vi "Execute.vi"(8 "error in (no error)":errorcluster, 9 "Workspace":T1, 10 "Cluster":T2, 11 "Pick and Place in":refnum<class "Pick and Place.lvclass">) -> (0 "error out":errorcluster, 2 "Control Out":T2, 3 "Pick and Place out":refnum<class "Pick and Place.lvclass">)   [LabVIEW 2020, in "Pick and Place.lvclass"]
uses:
  Pick and Place.lvclass
  Controller/Controllers.ctl
  Controller/I-O/I-O.lvclass
  Controller/Dispenser/Dispenser.lvclass
  C:/Program Files (x86)/Aerotech/A3200/LabVIEW/2010/Bin/Aerotech.A3200.dll
  Program Files (x86)/Aerotech/A3200/LabVIEW/2010/Bin/Aerotech.A3200.dll
  Workspace/Workspace.ctl
  Pick and Place.lvclass/Pick and Place.ctl
  686f831b-46dc-4046-ae8d-e6191224ee14.vi
  Controller/Motion/Motion.lvclass
  Controller/Motion/A3200/A3200.lvclass
  Controller/Controller.lvclass
  Workspace/Fixture.lvclass
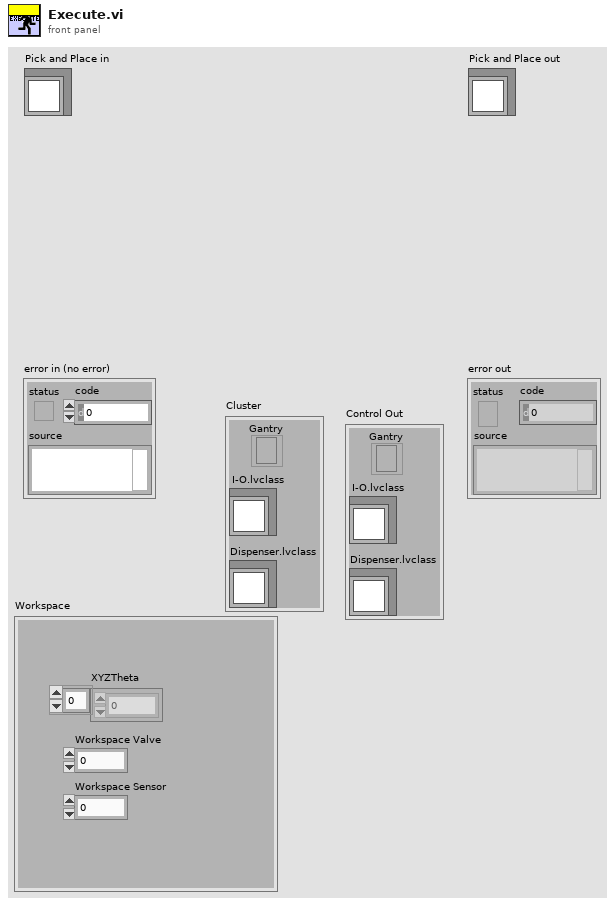
[diagram p1: front panel]
types:
  T1 = typedef "Fixture.lvclass/Workspace.ctl" = cluster{"XYZTheta":dbl[], "Workspace Valve":i32, "Workspace Sensor":i32}
  T2 = typedef "Controller.lvclass/Controllers.ctl" = cluster{"I-O.lvclass":refnum<class "I-O.lvclass">, "Dispenser.lvclass":refnum<class "Dispenser.lvclass">, "Gantry":refnum<k24>}
  T3 = typedef "Pick and Place.lvclass/Pick and Place Type.ctl" = enum16{"Primary Pick Up", "Secondary Pick Up", "Put Down All", "Pick Up All", "Put Down Secondary"}
  T4 = typedef "I-O.lvclass/Pin Map.ctl" = cluster{"Region Valves":i32[], "Extra Valves":dbl[][][], "Tool Primary Valve":i32, "Tool Secondary Valve":i32, "Region Sensors":i32[], "Extra Sensors":dbl[][][], "Tool Primary Sensor":dbl, "Tool Secondary Sensor":dbl, "Compression Sensor":dbl, "5V":i32}
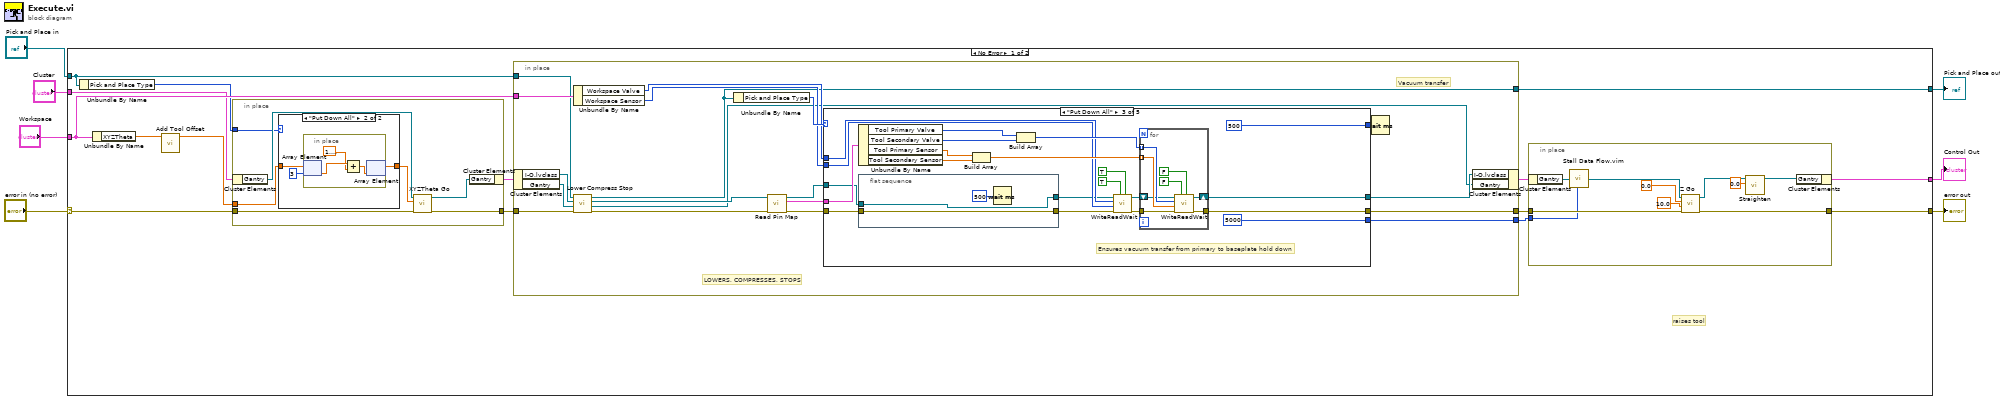
[diagram p0: block diagram]
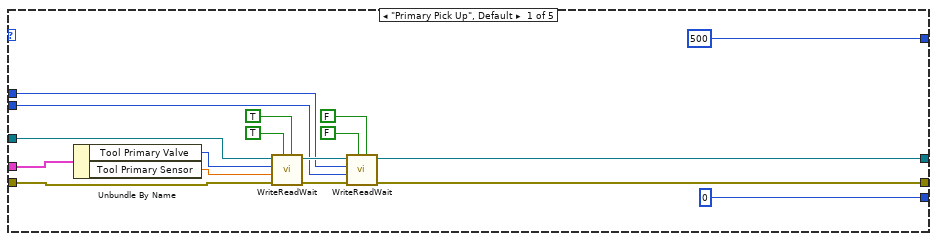
[diagram p2: hidden frame]
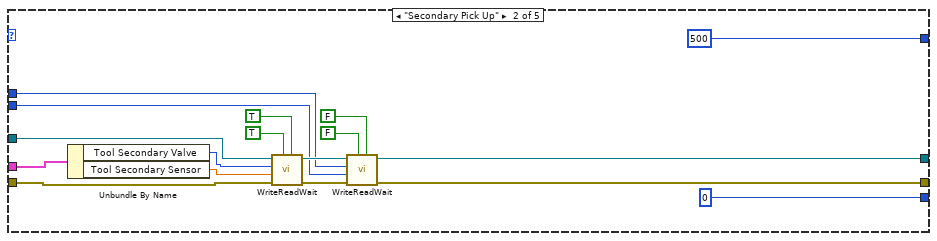
[diagram p3: hidden frame]
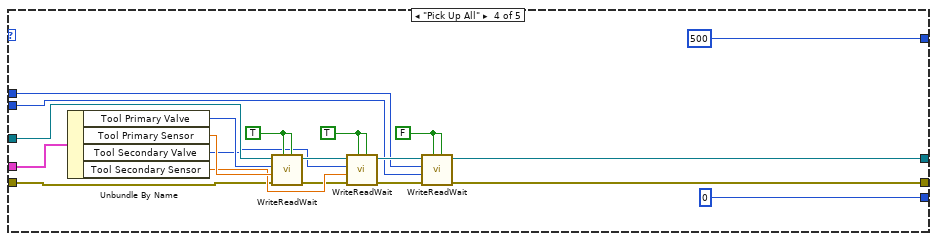
[diagram p4: hidden frame]
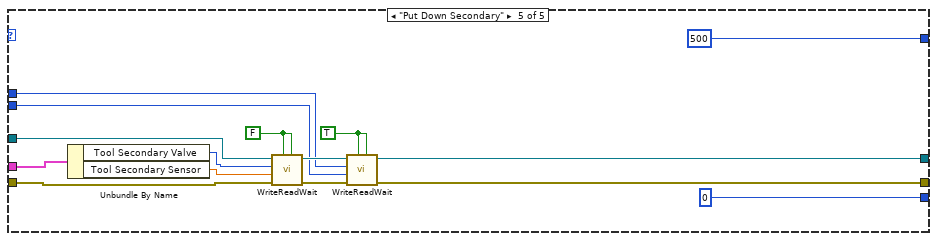
[diagram p5: hidden frame]
diagram:
  n1 = case shown="No Error" "error in (no error)" {
    selector: "error in (no error)" -> [w16 w168]
    tunnel: "Cluster" -> [w20 w169]
    tunnel: "Workspace" -> [w21 _]
    tunnel: [w15 w168] -> w1
    tunnel: [w19 w169] -> w2
    tunnel: "Pick and Place in" -> [w9 w167]
    tunnel: [w18 w167] -> w6
    frame No Error {
      # "raises tool"
      n2 = Unbundle By Name(w9) -> ("Pick and Place Type"=w8:T3)
      n3 = Unbundle By Name(w21) -> ("XYZTheta"=w13:dbl[])
      n4 = call "Add Tool Offset.vi"("XYZTheta"=w13) -> ("Array"=w17:dbl[])  [unwired: 10 in]
      n5 = in-place {
        in-place-border: w17 -> [w154]
        in-place-border: w16 -> [w156]
        in-place-border: [w157] -> w12
        in-place-border: w8 -> [w155]
        n6 = in-place-cluster #1(w20) -> ("Gantry"=w159:refnum<k24>)
        n7 = case shown="\"Put Down All\"" w155 {
          tunnel: w154 -> [w160 w163]
          tunnel: [w160 w161] -> w153
          frame "Primary Pick Up", Default {
          }
          frame "Put Down All" {
            n8 = in-place {
              n9 = in-place-array #2(w163, 3) -> (w166:dbl)
              n10 = Add(x=w166, y=1.5707963267948966) -> (x+y=w164:dbl)
              n11 = in-place-array #2(w164) -> (w161:dbl[])  [unwired: 1 out]
            }
          }
        }
        n12 = call "XYZTheta Go.vi"("error in (no error)"=w156, "XYZTheta In"=w153, "Gantry 2"=w159) -> ("error out"=w157:errorcluster, "Gantry 3"=w158:refnum<k24>)  [unwired: 6 in, 1 out]
        n13 = in-place-cluster #1("Gantry"=w158) -> (w22:T2)
      }
      n14 = in-place {
        in-place-border: w21 -> [w51]
        in-place-border: w9 -> [w41]
        in-place-border: [w40] -> w18
        in-place-border: w12 -> [w35]
        in-place-border: [w34] -> w11
        in-place-border: [w33] -> w10
        # "Vacuum transfer"
        # "LOWERS, COMPRESSES, STOPS"
        n15 = in-place-cluster #3(w22) -> ("I-O.lvclass"=w44:refnum<class "I-O.lvclass">, "Gantry"=w39:refnum<k24>)
        n16 = Unbundle By Name(w51) -> ("Workspace Valve"=w49:i32, "Workspace Sensor"=w48:i32)
        n17 = call "Lower Compress Stop.vi"("error in (no error)"=w35, "Gantry In"=w39, "I-O.lvclass"=w44, "Pick and Place in"=w41) -> ("error out"=w37:errorcluster, "Gantry Out"=w38:refnum<k24>, "I-O out"=w42:refnum<class "I-O.lvclass">, "Pick and Place Out"=w40:refnum<class "Pick and Place.lvclass">)  [unwired: 4 in]
        n18 = Unbundle By Name(w40) -> ("Pick and Place Type"=w50:T3)
        n19 = call-dynamic "Read Pin Map.vi"("error in (no error)"=w37, "I-O in"=w42) -> ("error out"=w36:errorcluster, "Pin Map 2"=w46:T4, "I-O out"=w45:refnum<class "I-O.lvclass">)  [unwired: 7 in]
        n20 = case shown="\"Put Down All\"" w50 {
          tunnel: w49 -> [w65 w77 w96 w127 w146]
          tunnel: w48 -> [w64 w76 w95 w126 w145]
          tunnel: [w59 w75 w100 w124 w143] -> w43
          tunnel: [u32 500 ("milliseconds to wait") 500 500 u32 500 ("milliseconds to wait") u32 500 ("milliseconds to wait")] -> w47
          tunnel: w45 -> [w58 w74 w91 w136 w151]
          tunnel: w46 -> [w57 w73 w94 w137 w152]
          tunnel: w36 -> [w55 w72 w88 w122 w141]
          tunnel: [w53 w70 w87 w119 w139] -> w34
          tunnel: [0 0 5000 0 0] -> w33
          frame "Primary Pick Up", Default {
            n21 = Unbundle By Name(w57) -> ("Tool Primary Valve"=w56:i32, "Tool Primary Sensor"=w67:dbl)
            n22 = call "WriteReadWait.vi"("Read Value"=TRUE, "Write Value"=TRUE, "error in (no error)"=w55, "Read"=w67, "Write"=w56, "I-O in"=w58) -> ("error out"=w54:errorcluster, "I-O out"=w66:refnum<class "I-O.lvclass">)  [unwired: 4 in]
            n23 = call "WriteReadWait.vi"("Read Value"=FALSE ("Write Value"), "Write Value"=FALSE ("Read Value"), "error in (no error)"=w54, "Read"=w64, "Write"=w65, "I-O in"=w66) -> ("error out"=w53:errorcluster, "I-O out"=w59:refnum<class "I-O.lvclass">)  [unwired: 4 in]
          }
          frame "Secondary Pick Up" {
            n24 = Unbundle By Name(w73) -> ("Tool Secondary Valve"=w79:i32, "Tool Secondary Sensor"=w78:dbl)
            n25 = call "WriteReadWait.vi"("Read Value"=TRUE, "Write Value"=TRUE, "error in (no error)"=w72, "Read"=w78, "Write"=w79, "I-O in"=w74) -> ("error out"=w71:errorcluster, "I-O out"=w84:refnum<class "I-O.lvclass">)  [unwired: 4 in]
            n26 = call "WriteReadWait.vi"("Read Value"=FALSE ("Write Value"), "Write Value"=FALSE ("Read Value"), "error in (no error)"=w71, "Read"=w76, "Write"=w77, "I-O in"=w84) -> ("error out"=w70:errorcluster, "I-O out"=w75:refnum<class "I-O.lvclass">)  [unwired: 4 in]
          }
          frame "Put Down All" {
            # "Ensures vacuum transfer from primary to baseplate hold down"
            n27 = Unbundle By Name(w94) -> ("Tool Primary Valve"=w101:i32, "Tool Secondary Valve"=w102:i32, "Tool Primary Sensor"=w103:dbl, "Tool Secondary Sensor"=w104:dbl)
            n28 = flat-sequence {
              tunnel: [w108] -> w92
              tunnel: w91 -> [w108]
              tunnel: [w107] -> w89
              tunnel: w88 -> [w107]
              frame #0 {
                # "Delay After Placing"
                n29 = Wait (ms)(milliseconds to wait=u32 500) -> ()  [unwired: 1 out]
              }
            }
            n30 = Build Array(w103, w104) -> (w106:dbl[])
            n31 = Build Array(w101, w102) -> (w105:i32[])
            n32 = call "WriteReadWait.vi"("Read Value"=TRUE, "Write Value"=TRUE, "error in (no error)"=w89, "Read"=w95, "Write"=w96, "I-O in"=w92) -> ("error out"=w90:errorcluster, "I-O out"=w93:refnum<class "I-O.lvclass">)  [unwired: 4 in]
            n33 = for {
              shift-right: [w112] -> w100
              shift-left: w93 -> [w113]
              tunnel: w105 -> [w115] mode=indexing
              tunnel: w106 -> [w114] mode=indexing
              tunnel: w90 -> [w111]
              tunnel: [w110] -> w87
              n34 = call "WriteReadWait.vi"("Read Value"=FALSE ("Write Value"), "Write Value"=FALSE ("Read Value"), "error in (no error)"=w111, "Read"=w114, "Write"=w115, "I-O in"=w113) -> ("error out"=w110:errorcluster, "I-O out"=w112:refnum<class "I-O.lvclass">)  [unwired: 4 in]
            }
          }
          frame "Pick Up All" {
            w125 = FALSE ("Read Value")
            w129 = TRUE ("Write Value")
            w135 = TRUE ("Write Value")
            n35 = Unbundle By Name(w137) -> ("Tool Primary Valve"=w134:i32, "Tool Primary Sensor"=w133:dbl, "Tool Secondary Valve"=w131:i32, "Tool Secondary Sensor"=w130:dbl)
            n36 = call "WriteReadWait.vi"("Read Value"=w135, "Write Value"=w135, "error in (no error)"=w122, "Read"=w133, "Write"=w134, "I-O in"=w136) -> ("error out"=w121:errorcluster, "I-O out"=w132:refnum<class "I-O.lvclass">)  [unwired: 4 in]
            n37 = call "WriteReadWait.vi"("Read Value"=w129, "Write Value"=w129, "error in (no error)"=w121, "Read"=w130, "Write"=w131, "I-O in"=w132) -> ("error out"=w120:errorcluster, "I-O out"=w128:refnum<class "I-O.lvclass">)  [unwired: 4 in]
            n38 = call "WriteReadWait.vi"("Read Value"=w125, "Write Value"=w125, "error in (no error)"=w120, "Read"=w126, "Write"=w127, "I-O in"=w128) -> ("error out"=w119:errorcluster, "I-O out"=w124:refnum<class "I-O.lvclass">)  [unwired: 4 in]
          }
          frame "Put Down Secondary" {
            w144 = TRUE ("Read Value")
            w148 = FALSE ("Write Value")
            n39 = Unbundle By Name(w152) -> ("Tool Secondary Valve"=w150:i32, "Tool Secondary Sensor"=w149:dbl)
            n40 = call "WriteReadWait.vi"("Read Value"=w148, "Write Value"=w148, "error in (no error)"=w141, "Read"=w149, "Write"=w150, "I-O in"=w151) -> ("error out"=w140:errorcluster, "I-O out"=w147:refnum<class "I-O.lvclass">)  [unwired: 4 in]
            n41 = call "WriteReadWait.vi"("Read Value"=w144, "Write Value"=w144, "error in (no error)"=w140, "Read"=w145, "Write"=w146, "I-O in"=w147) -> ("error out"=w139:errorcluster, "I-O out"=w143:refnum<class "I-O.lvclass">)  [unwired: 4 in]
          }
        }
        n42 = Wait (ms)(milliseconds to wait=w47) -> ()  [unwired: 1 out]
        n43 = in-place-cluster #3("I-O.lvclass"=w43, "Gantry"=w38) -> (w14:T2)
      }
      n44 = in-place {
        in-place-border: [w30] -> w15
        in-place-border: w11 -> [w29]
        in-place-border: w10 -> [w26]
        n45 = in-place-cluster #4(w14) -> ("Gantry"=w28:refnum<k24>)
        n46 = call "Stall Data Flow.vim"("value in"=w28, "milliseconds to wait"=w26) -> ("value out"=w27:refnum<k24>)  [unwired: 1 out]
        n47 = call "Z Go.vi"("error in (no error)"=w29, "Speed"=10.0 ("speed"), "Position"=0.0 ("position"), "Gantry 2"=w27) -> ("error out"=w30:errorcluster, "Gantry 3"=w25:refnum<k24>)  [unwired: 6 in]
        n48 = call "Straighten.vi"("Angle (rad)"=0.0, "Gantry 2"=w25) -> ("Gantry 3"=w24:refnum<k24>)  [unwired: 8 in, 1 out]
        n49 = in-place-cluster #4("Gantry"=w24) -> (w19:T2)
      }
    }
    frame Error {
    }
  }
  "error out" <- w1
  "Pick and Place out" <- w6
  "Control Out" <- w2
